vi "Migrate Measurement Dependencies.vi"(0 "Project path":path, 5 "Measurement path":path, 7 "Dependencies path":path[](array[path]), 9 "Plug-in name":string, 11 "error in (no error)":errorcluster) -> (4 "Project reference":refnum<vi>, 6 "MeasurementCore reference":refnum<vi>, 8 "Outside items":string[](array[string]), 15 "error out":errorcluster)   [LabVIEW 2021]
uses:
  controls/Library Info.ctl
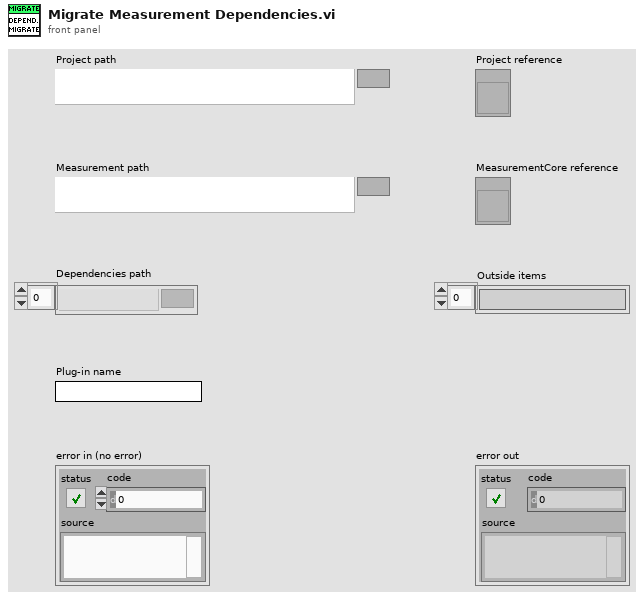
[diagram p1: front panel]
types:
  T1 = typedef "Library Info.ctl" = cluster{"Library path":path, "Library name":string}
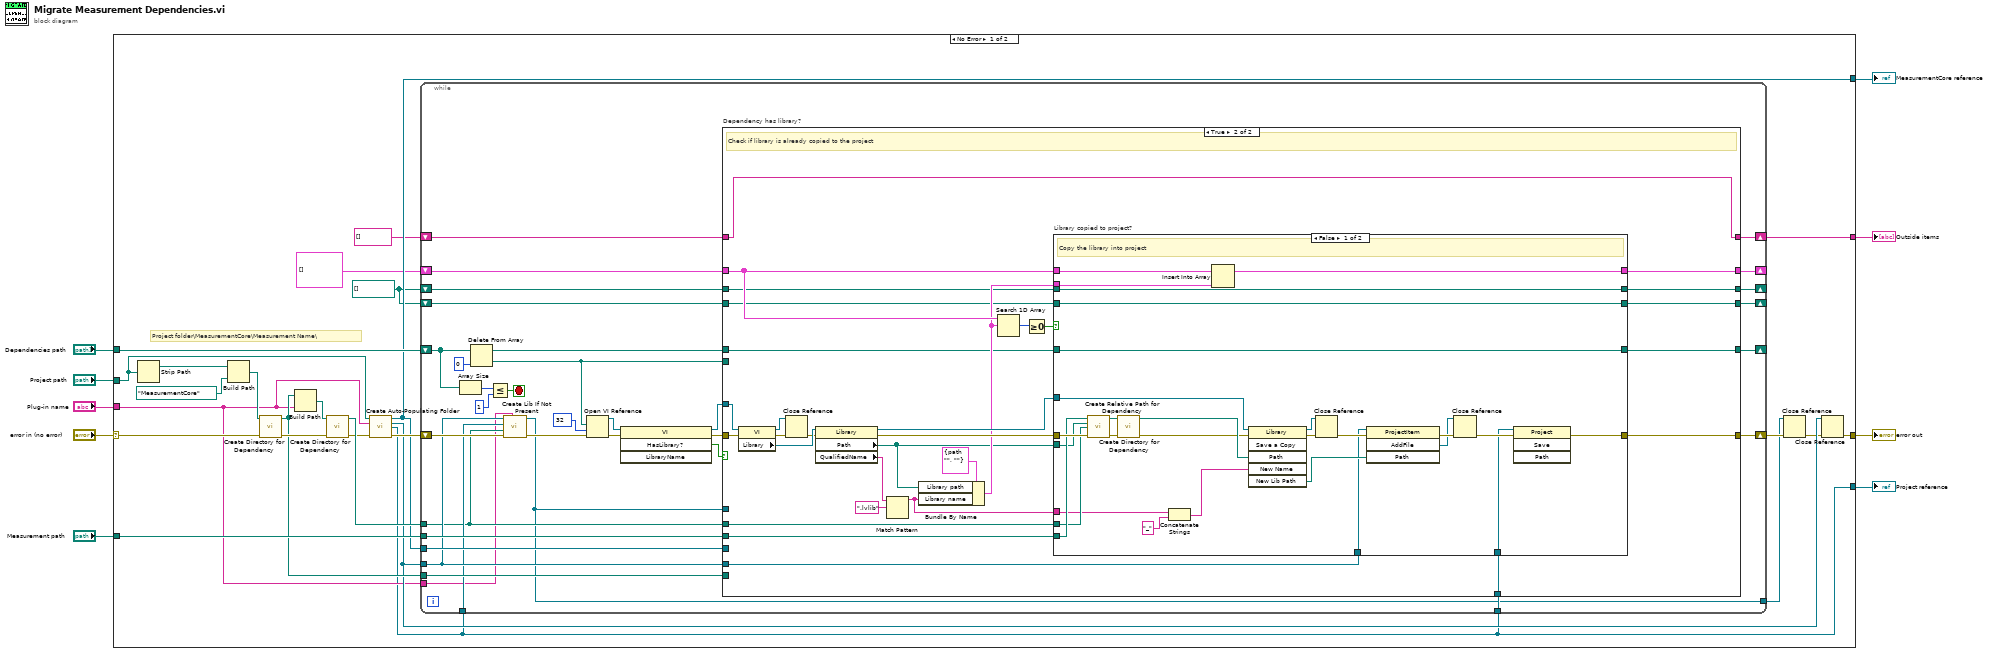
[diagram p0: block diagram]
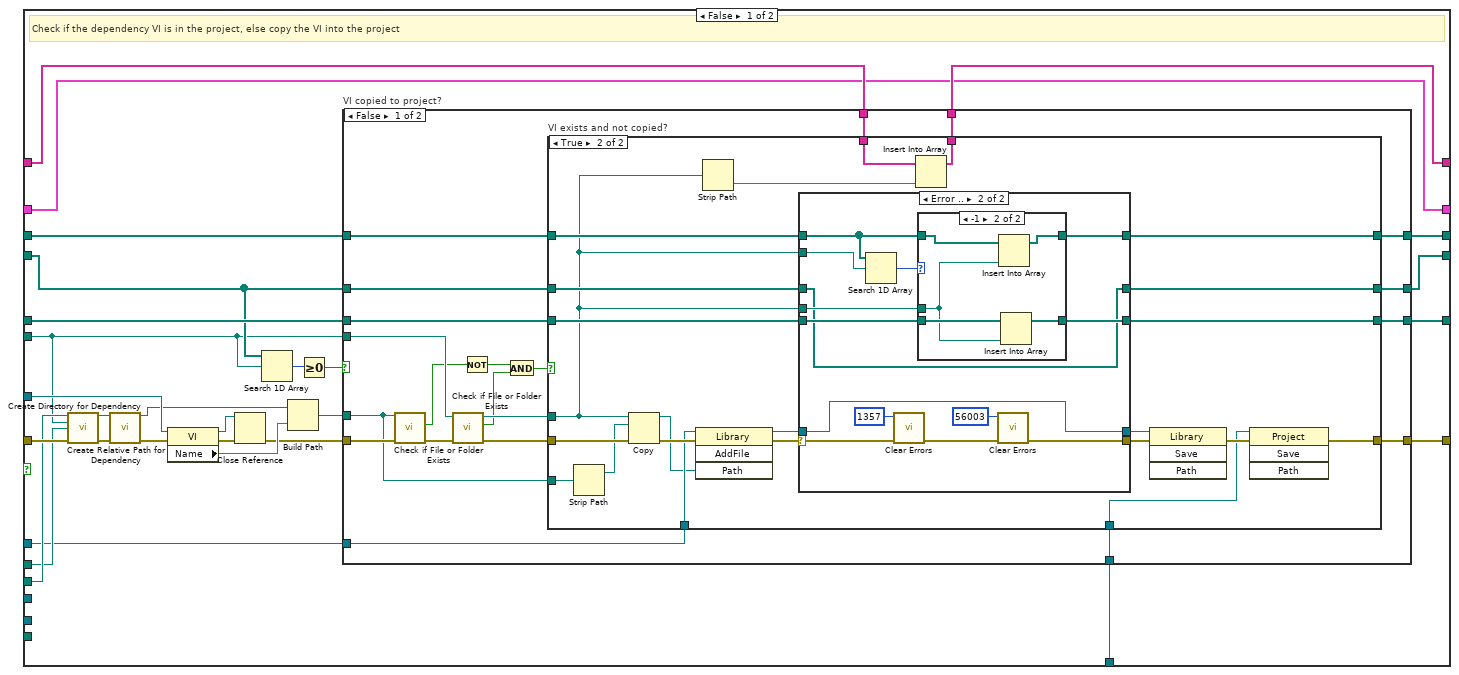
[diagram p2: hidden frame]
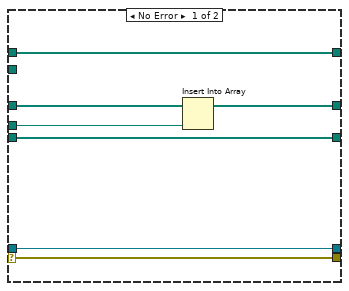
[diagram p4: hidden frame]
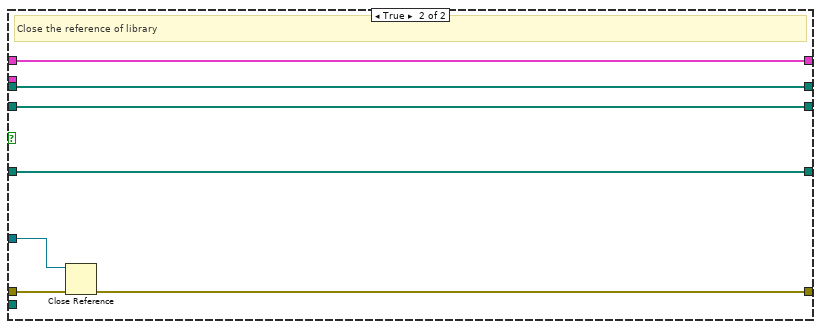
[diagram p7: hidden frame]
diagram:
  n1 = case shown="No Error" "error in (no error)" {
    selector: "error in (no error)" -> [w26 w244]
    tunnel: [w19 w244] -> w8
    tunnel: "Project path" -> [w25 _]
    tunnel: "Measurement path" -> [w30 _]
    tunnel: "Dependencies path" -> [w34 _]
    tunnel: "Plug-in name" -> [w17 _]
    tunnel: [w21 _] -> w3
    tunnel: [w14 _] -> w2
    tunnel: [w15 _] -> w1
    frame No Error {
      w10 = path[] []
      # "Project folder\\MeasurementCore\\Measurement Name\\"
      n2 = Strip Path(path=w25) -> (stripped path=w29:path)  [unwired: 1 out]
      n3 = Build Path(base path=w29, name or relative path=path "MeasurementCore") -> (appended path=w27:path)
      n4 = call "Create Directory for Dependency.vi"("Directory path"=w27, "error in (no error)"=w26) -> ("Directory path out"=w20:path, "error out"=w24:errorcluster)  [unwired: 12 in]
      n5 = Build Path(base path=w20, name or relative path=w17) -> (appended path=w33:path)
      n6 = call "Create Directory for Dependency.vi"("Directory path"=w33, "error in (no error)"=w24) -> ("Directory path out"=w32:path, "error out"=w23:errorcluster)  [unwired: 12 in]
      n7 = call "Create Auto-Populating Folder.vi"("Project path"=w25, "Plug-in name"=w17, "error in (no error)"=w23) -> ("MeasurementCore reference"=w21:refnum<vi>, "Folder reference"=w18:refnum<vi>, "Project reference"=w14:refnum<vi>, "error out"=w22:errorcluster)  [unwired: 9 in]
      n8 = while {
        shift-right: [w56] -> w31
        shift-left: w22 -> [w44]
        shift-right: [w49] -> _
        shift-left: w34 -> [w66]
        tunnel: w32 -> [w40]
        shift-right: [w55] -> _
        shift-left: T1[] [] -> [w58]
        tunnel: w30 -> [w54]
        shift-right: [w51] -> _
        shift-left: w10 -> [w52]
        tunnel: w21 -> [w48]
        tunnel: w20 -> [w47]
        tunnel: w18 -> [w42]
        tunnel: w17 -> [w39]
        shift-right: [w45] -> w15
        shift-left: string[] [] -> [w46]
        tunnel: w14 -> [w41]
        tunnel: w14 -> [w38]
        shift-right: [w37] -> _
        shift-left: w10 -> [w36]
        tunnel: [w35] -> w12
        stop <- w65 stop-if-true
        n9 = Array Size(array=w66) -> (size(s)=w68:i32)
        n10 = Delete From Array(array=w66, index=0) -> (deleted portion=w53:path, array with subset deleted=w50:path[])  [unwired: 1 in]
        n11 = Less Or Equal?(x=w68, y=1) -> (x <= y?=w65:bool)
        n12 = call "Create Lib If Not Present.vi"("Plug-in name"=w39, "error in (no error)"=w44, "DestDirectory"=w40, "ProjectRef"=w41, "VirtualFolderRef"=w42) -> ("error out"=w43:errorcluster, "Library Refnum"=w35:refnum<vi>)  [unwired: 5 in]
        n13 = Open VI Reference(vi path=w53, options=32, error in (no error)=w43) -> (vi reference=w62:refnum<vi>, error out=w64:errorcluster)  [unwired: 3 in]
        n14 = invoke class="VI" method="HasLibrary?"(reference=w62, error in=w64) -> (reference out=w59:refnum<vi>, error out=w60:errorcluster, "Has Library?"=w61:bool)  [unwired: 2 in, 1 out]
        n15 = case "Dependency has library?" shown="True" w61 {
          tunnel: w60 -> [w95 w207]
          tunnel: w59 -> [w91 w208]
          tunnel: w58 -> [w72 w195]
          tunnel: [w86 w196] -> w56
          tunnel: [w72 w194] -> w55
          tunnel: w54 -> [w94 w192]
          tunnel: w40 -> [w77 w190]
          tunnel: w53 -> [w81 _]
          tunnel: w52 -> [w82 w187]
          tunnel: [w76 w186] -> w51
          tunnel: w50 -> [w85 w185]
          tunnel: [w84 w184] -> w49
          tunnel: w48 -> [_ _]
          tunnel: w47 -> [_ _]
          tunnel: w42 -> [_ w183]
          tunnel: w46 -> [w74 w182]
          tunnel: [w73 w182] -> w45
          tunnel: w35 -> [w75 _]
          tunnel: w38 -> [w69 w181]
          tunnel: [w71 w179] -> w37
          tunnel: w36 -> [w70 w180]
          frame False {
            # "Check if the dependency VI is in the project, else copy the VI into the project"
            n16 = call "Create Relative Path for Dependency.vi"("Old Main Path"=w94, "Old Dependency Path"=w81, "New Dir"=w77, "error in (no error)"=w95) -> ("Directory"=w93:path, "error out"=w96:errorcluster)  [unwired: 10 in]
            n17 = call "Create Directory for Dependency.vi"("Directory path"=w93, "error in (no error)"=w96) -> ("Directory path out"=w83:path, "error out"=w92:errorcluster)  [unwired: 12 in]
            n18 = property class="VI"(reference=w91, error in=w92) -> (reference out=w87:refnum<vi>, error out=w90:errorcluster, "Name"=w89:string)
            n19 = Close Reference(reference=w87, error in (no error)=w90) -> (error out=w88:errorcluster)
            n20 = Search 1D Array(1D array=w82, element=w81) -> (index of element=w80:i32)  [unwired: 1 in]
            n21 = Build Path(base path=w83, name or relative path=w89) -> (appended path=w79:path)
            n22 = Greater Or Equal To 0?(x=w80) -> (x >= 0?=w78:bool)
            n23 = case "VI copied to project?" shown="False" w78 {
              tunnel: w88 -> [w117 w178]
              tunnel: w81 -> [w116 _]
              tunnel: [w113 w178] -> w86
              tunnel: w82 -> [w112 w177]
              tunnel: [w111 w177] -> w76
              tunnel: w79 -> [w107 _]
              tunnel: w85 -> [w110 w176]
              tunnel: [w109 w176] -> w84
              tunnel: w74 -> [w102 w175]
              tunnel: [w101 w175] -> w73
              tunnel: w75 -> [w100 _]
              tunnel: [w99 w174] -> w71
              tunnel: w70 -> [w98 w174]
              tunnel: w69 -> [w97 _]
              frame False {
                n24 = call <vilib>:"Check if File or Folder Exists.vi"("error in (no error)"=w117, "path"=w107) -> ("error out"=w108:errorcluster, "file or folder exists?"=w106:bool)  [unwired: 7 in, 1 out]
                n25 = call <vilib>:"Check if File or Folder Exists.vi"("error in (no error)"=w108, "path"=w116) -> ("error out"=w115:errorcluster, "file or folder exists?"=w104:bool, "dup path"=w114:path)  [unwired: 7 in]
                n26 = Not(x=w106) -> (.not. x?=w105:bool)
                n27 = And(x=w105, y=w104) -> (x .and. y?=w103:bool)
                n28 = case "VI exists and not copied?" shown="True" w103 {
                  tunnel: w115 -> [w122 w145]
                  tunnel: w114 -> [_ w123]
                  tunnel: [w122 w125] -> w113
                  tunnel: w112 -> [w121 w144]
                  tunnel: [w121 w143] -> w111
                  tunnel: w107 -> [_ w139]
                  tunnel: w110 -> [w120 w127]
                  tunnel: [w120 w126] -> w109
                  tunnel: w102 -> [w119 w138]
                  tunnel: [w119 w136] -> w101
                  tunnel: w100 -> [_ w135]
                  tunnel: [w118 w133] -> w99
                  tunnel: w98 -> [w118 w132]
                  tunnel: w97 -> [_ w124]
                  frame False {
                  }
                  frame True {
                    n29 = Strip Path(path=w139) -> (stripped path=w141:path)  [unwired: 1 out]
                    n30 = Copy(8:w145, 10:w141, 11:w123) -> (0:w142:errorcluster, 3:w134:path)  [unwired: 2 in, 1 out]
                    n31 = invoke class="Library" method="AddFile"(reference=w135, error in=w142, "Path"=w134) -> (reference out=w131:refnum<vi>, error out=w130:errorcluster)  [unwired: 1 in, 2 out]
                    n32 = Strip Path(path=w123) -> (name=w137:string)  [unwired: 1 out]
                    n33 = case shown="Error .." w130 {
                      selector: w130 -> [w147 w166]
                      tunnel: w144 -> [w152 w153]
                      tunnel: [w151 w153] -> w143
                      tunnel: w123 -> [w150 w156]
                      tunnel: [w149 w157] -> w133
                      tunnel: w132 -> [w149 w158]
                      tunnel: [w148 w155] -> w128
                      tunnel: w131 -> [w148 w155]
                      tunnel: [w147 w164] -> w129
                      tunnel: w127 -> [w146 w160]
                      tunnel: [w146 w159] -> w126
                      tunnel: w123 -> [_ w161]
                      frame No Error {
                        n34 = Insert Into Array(array=w152, new element=w150) -> (w151:path[])  [unwired: 1 in]
                      }
                      frame Error {
                        n35 = Search 1D Array(1D array=w158, element=w161) -> (index of element=w154:i32)  [unwired: 1 in]
                        n36 = call <vilib>:"Clear Errors.vi"("error in (no error)"=w166, "specific error code to clear (0: all)"=1357) -> ("error out"=w165:errorcluster)  [unwired: 4 in, 1 out]
                        n37 = case shown="-1" w154 {
                          tunnel: w160 -> [w167 w173]
                          tunnel: [w167 w172] -> w159
                          tunnel: w158 -> [w168 w171]
                          tunnel: [w168 w170] -> w157
                          tunnel: w156 -> [_ w169]
                          frame Default {
                          }
                          frame -1 {
                            n38 = Insert Into Array(array=w171, new element=w169) -> (w170:path[])  [unwired: 1 in]
                            n39 = Insert Into Array(array=w173, new element=w169) -> (w172:path[])  [unwired: 1 in]
                          }
                        }
                        n40 = call <vilib>:"Clear Errors.vi"("error in (no error)"=w165, "specific error code to clear (0: all)"=56003) -> ("error out"=w164:errorcluster)  [unwired: 4 in, 1 out]
                      }
                    }
                    n41 = Insert Into Array(array=w138, new element=w137) -> (w136:string[])  [unwired: 1 in]
                    n42 = invoke class="Library" method="Save"(reference=w128, error in=w129) -> (error out=w140:errorcluster)  [unwired: 2 in, 3 out]
                    n43 = invoke class="Project" method="Save"(reference=w124, error in=w140) -> (error out=w125:errorcluster)  [unwired: 2 in, 3 out]
                  }
                }
              }
              frame True {
              }
            }
          }
          frame True {
            # "Check if library is already copied to the project"
            n44 = property class="VI"(reference=w208, error in=w207) -> (reference out=w198:refnum<vi>, error out=w206:errorcluster, "Library"=w205:refnum<vi>)
            n45 = Close Reference(reference=w198, error in (no error)=w206) -> (error out=w199:errorcluster)
            n46 = property class="Library"(reference=w205, error in=w199) -> (reference out=w197:refnum<vi>, error out=w200:errorcluster, "Path"=w191:path, "QualifiedName"=w201:string)
            n47 = Match Pattern(string=w201, regular expression=".lvlib") -> (before substring=w188:string)  [unwired: 1 in, 3 out]
            n48 = Bundle By Name(cluster=T1 {"Library path"=path "", "Library name"=""} ("Cluster"), "Library path"=w191, "Library name"=w188) -> (w193:T1)
            n49 = Search 1D Array(1D array=w195, element=w193) -> (index of element=w203:i32)  [unwired: 1 in]
            n50 = Greater Or Equal To 0?(x=w203) -> (x >= 0?=w202:bool)
            n51 = case "Library copied to project?" shown="False" w202 {
              tunnel: w200 -> [w231 w242]
              tunnel: w197 -> [w224 w243]
              tunnel: [w211 w241] -> w196
              tunnel: w195 -> [w236 w240]
              tunnel: [w235 w240] -> w194
              tunnel: w193 -> [w234 _]
              tunnel: w192 -> [w230 _]
              tunnel: w191 -> [w229 _]
              tunnel: w190 -> [w228 _]
              tunnel: w188 -> [w214 _]
              tunnel: w187 -> [w221 w239]
              tunnel: [w221 w239] -> w186
              tunnel: [w220 w238] -> w184
              tunnel: w185 -> [w220 w238]
              tunnel: w183 -> [w215 _]
              tunnel: w181 -> [w210 _]
              tunnel: [w209 w237] -> w179
              tunnel: w180 -> [w209 w237]
              frame False {
                # "Copy the library into project"
                n52 = call "Create Relative Path for Dependency.vi"("Old Main Path"=w230, "Old Dependency Path"=w229, "New Dir"=w228, "error in (no error)"=w231) -> ("Directory"=w226:path, "error out"=w227:errorcluster)  [unwired: 10 in]
                n53 = call "Create Directory for Dependency.vi"("Directory path"=w226, "error in (no error)"=w227) -> ("Directory path out"=w225:path, "error out"=w223:errorcluster)  [unwired: 12 in]
                n54 = Concatenate Strings(w214, "_" ("string")) -> (w212:string)
                n55 = Insert Into Array(array=w236, new element=w234) -> (w235:T1[])  [unwired: 1 in]
                n56 = invoke class="Library" method="Save a Copy"(reference=w224, error in=w223, "Path"=w225, "New Name"=w212) -> (reference out=w232:refnum<vi>, error out=w233:errorcluster, "New Lib Path"=w218:path)  [unwired: 2 in, 3 out]
                n57 = Close Reference(reference=w232, error in (no error)=w233) -> (error out=w222:errorcluster)
                n58 = invoke class="ProjectItem" method="AddFile"(reference=w215, error in=w222, "Path"=w218) -> (error out=w219:errorcluster, "AddFile"=w216:refnum<vi>)  [unwired: 1 in, 2 out]
                n59 = Close Reference(reference=w216, error in (no error)=w219) -> (error out=w217:errorcluster)
                n60 = invoke class="Project" method="Save"(reference=w210, error in=w217) -> (error out=w211:errorcluster)  [unwired: 2 in, 3 out]
              }
              frame True {
                # "Close the reference of library"
                n61 = Close Reference(reference=w243, error in (no error)=w242) -> (error out=w241:errorcluster)
              }
            }
          }
        }
      }
      n62 = Close Reference(reference=w12, error in (no error)=w31) -> (error out=w13:errorcluster)
      n63 = Close Reference(reference=w18, error in (no error)=w13) -> (error out=w19:errorcluster)
    }
    frame Error {
    }
  }
  "error out" <- w8
  "MeasurementCore reference" <- w3
  "Project reference" <- w2
  "Outside items" <- w1
